vi "MNK_Dashboard_v2.vi"() -> ()   [LabVIEW 2013]
panel:
  out "magnet chart":dbl(graph)
  out "LN2 chart":dbl(graph)
  out "LHe chart":dbl(graph)
  out "temperature chart":dbl(graph)
  in  "Preferences Button":bool
  in  "OK":bool
  out "LN2 Level (mm)":dbl
  out "LHe Level (mm)":dbl
  out "Temperature (mK)":dbl format="%_3p"
  out "Magnetic Field (T)":dbl format="%.2f"
  # "magnetic field (T)"
  # "temperature (mK)"
  # "LHe level (mm)"
  # "LN2 level (mm)"
  # "hit \"enter\" to stop (on What Is)"
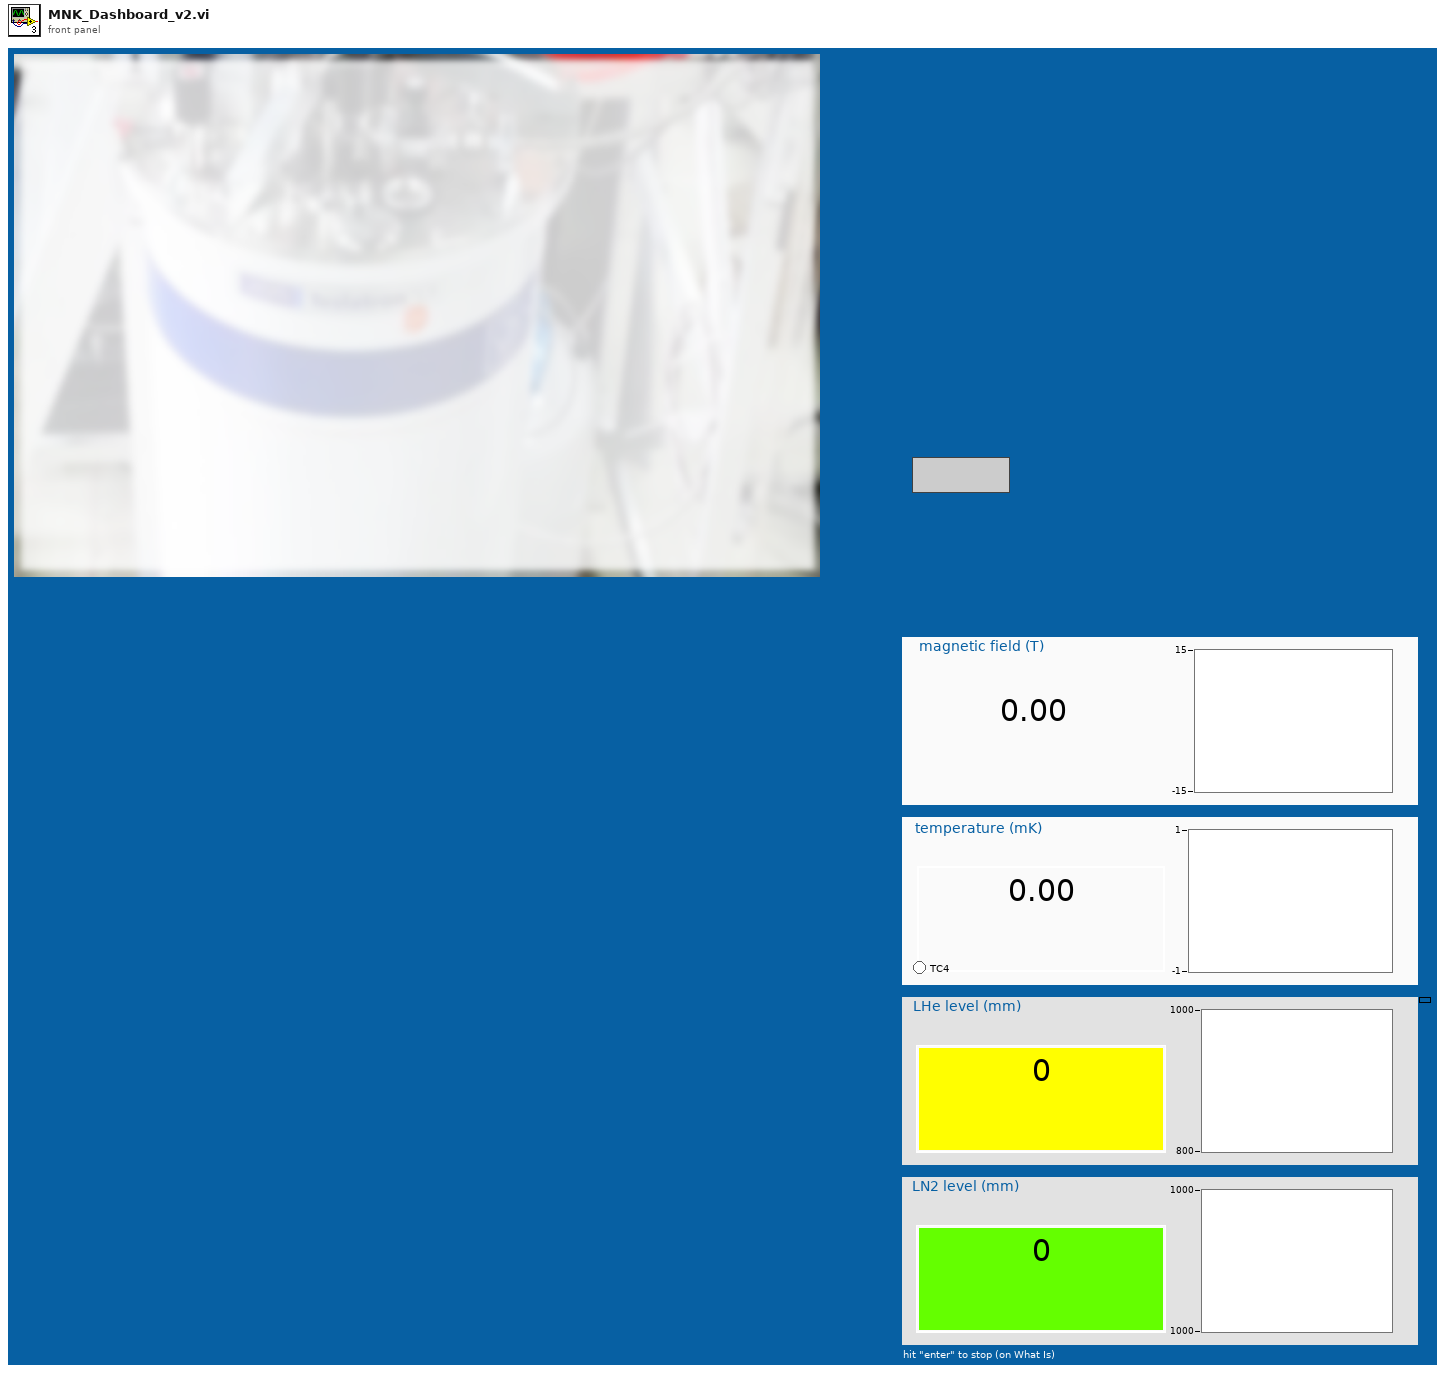
[diagram p1: front panel]
types:
  T1 = enum32{"invalid app kind", "Development System", "Run Time System", "Student Edition", "Embedded LabVIEW", "Evaluation", "Custom"}
  T2 = enum32{"Invalid", "Standard", "Closed", "Hidden", "Minimized", "Maximized"}
  T3 = cluster{"Core":cluster{"Current VI Reference":refnum<vi>, "Close Panel on Exit?":bool}, "Your Boolean data":bool, "Your string data":string}
  T4 = cluster{"Current VI Reference":refnum<vi>, "Close Panel on Exit?":bool}
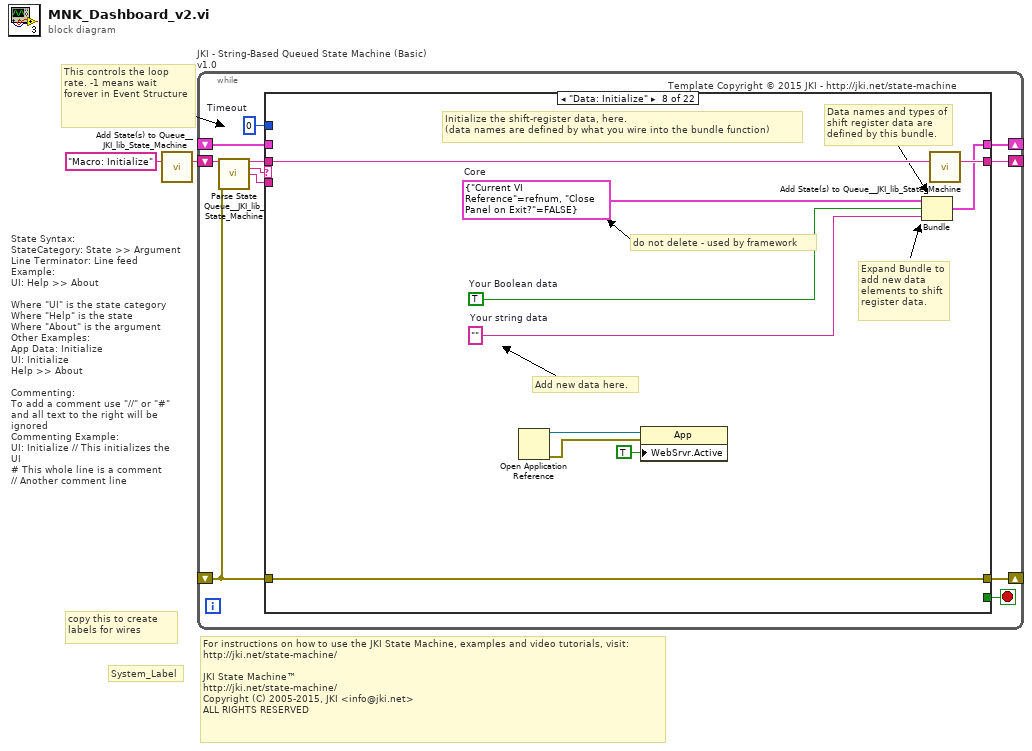
[diagram p0: block diagram]
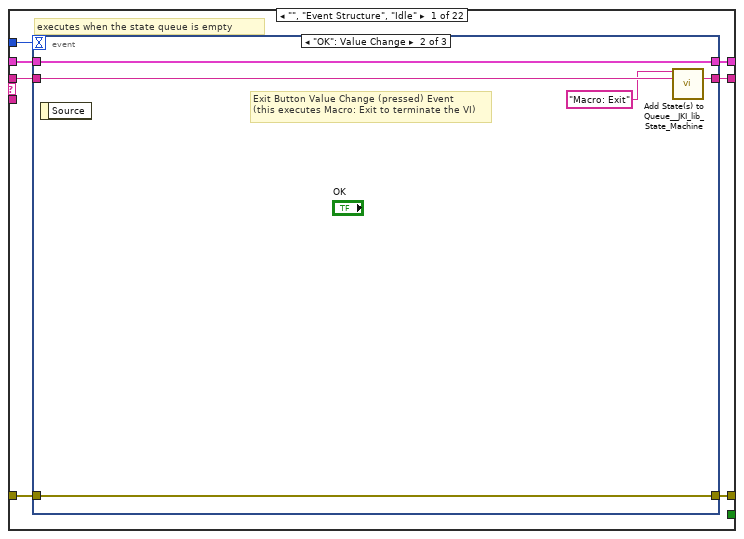
[diagram p2: hidden frame]
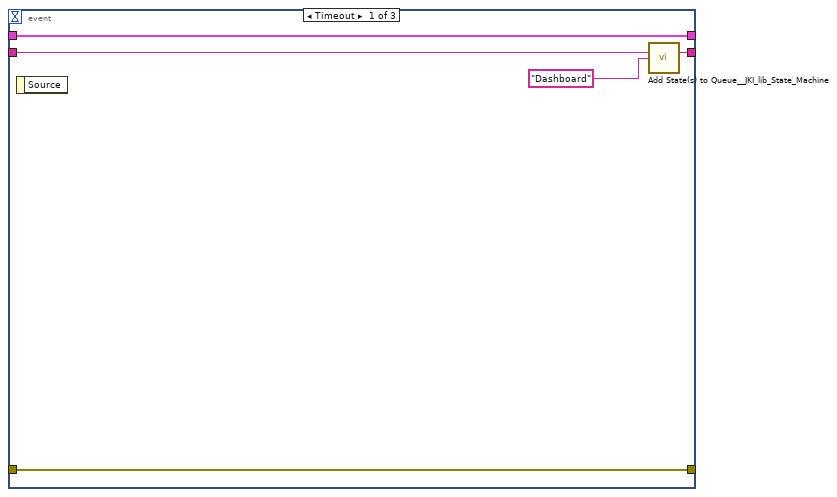
[diagram p3: hidden frame]
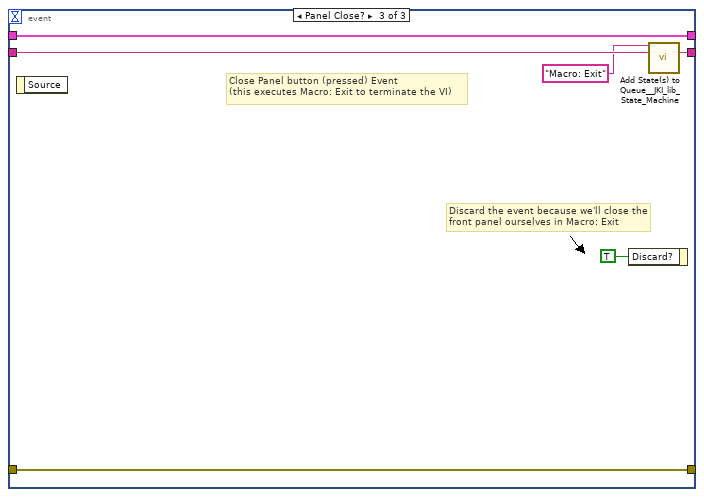
[diagram p4: hidden frame]
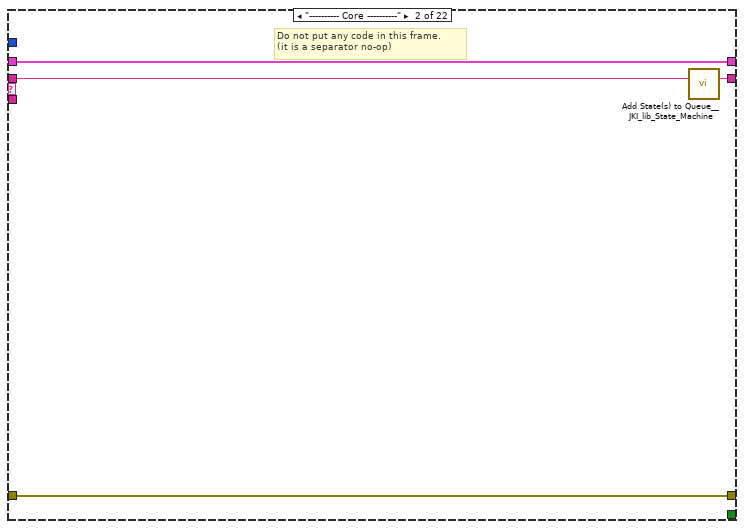
[diagram p5: hidden frame]
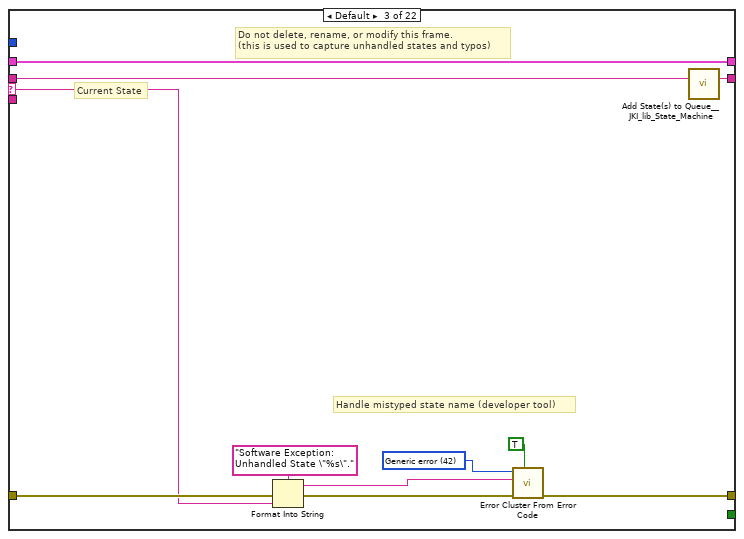
[diagram p6: hidden frame]
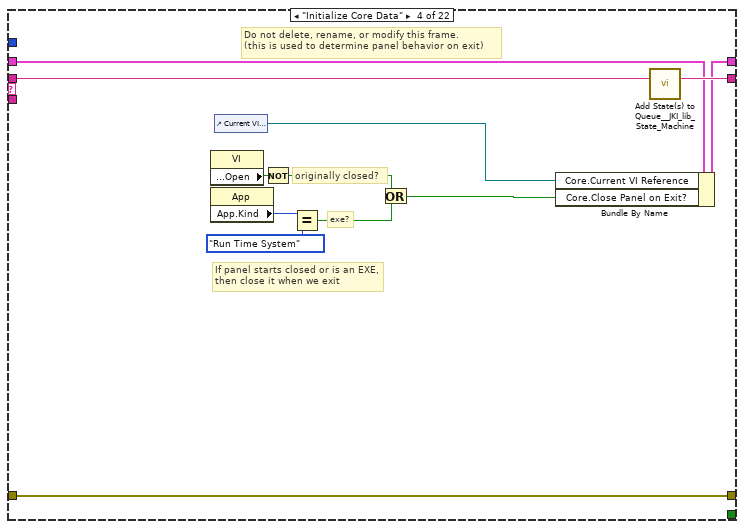
[diagram p7: hidden frame]
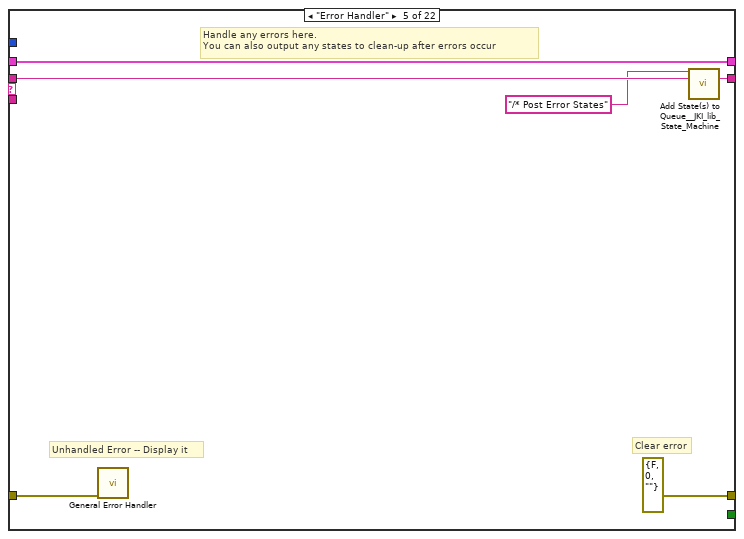
[diagram p8: hidden frame]
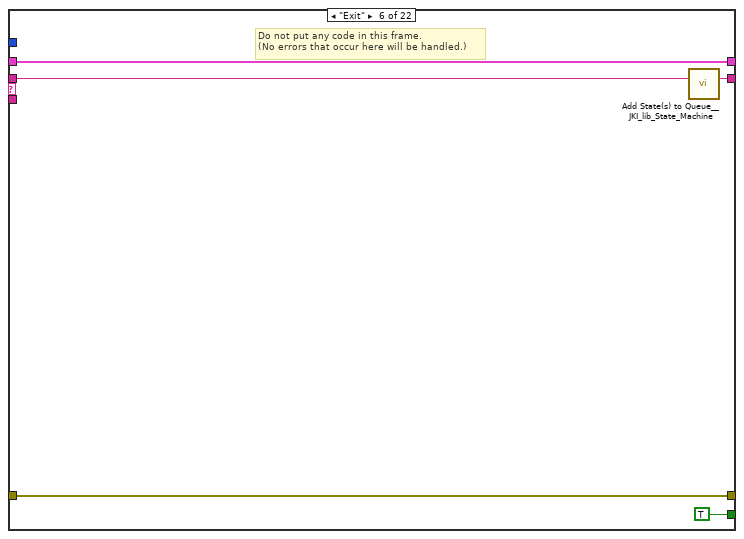
[diagram p9: hidden frame]
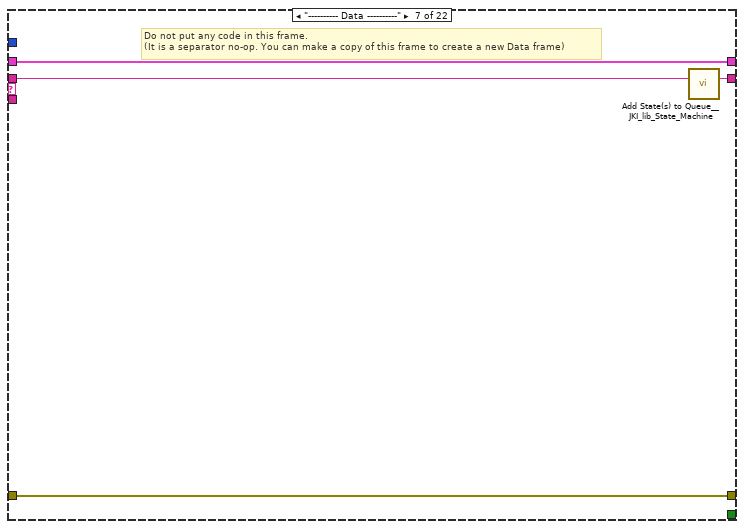
[diagram p10: hidden frame]
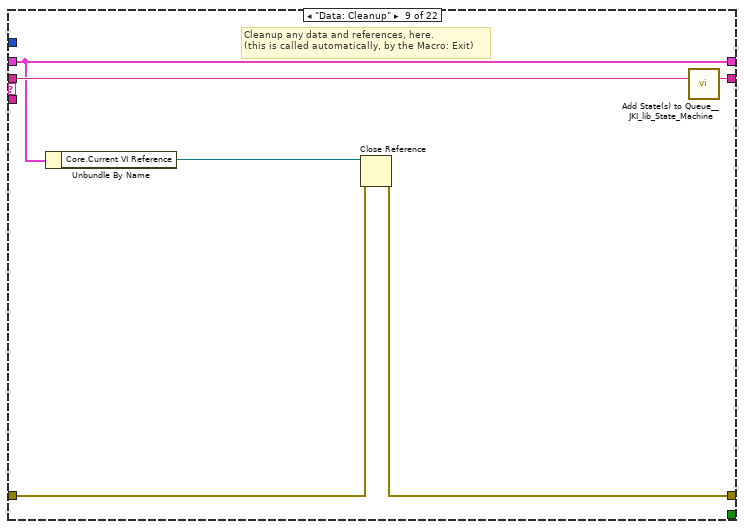
[diagram p11: hidden frame]
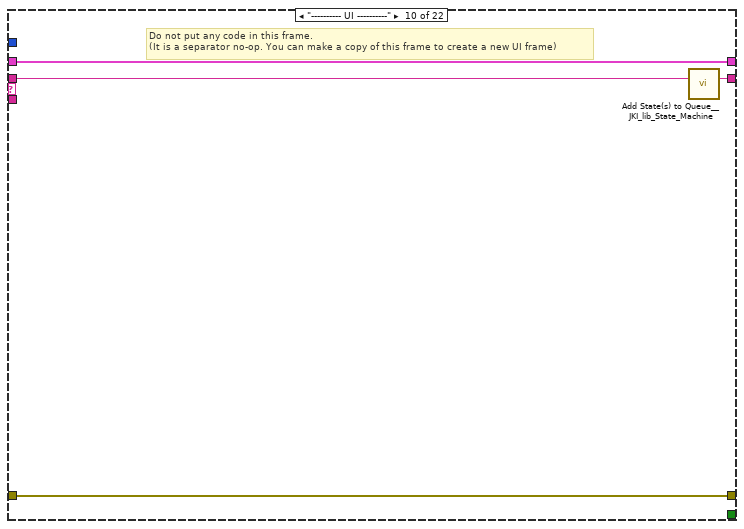
[diagram p12: hidden frame]
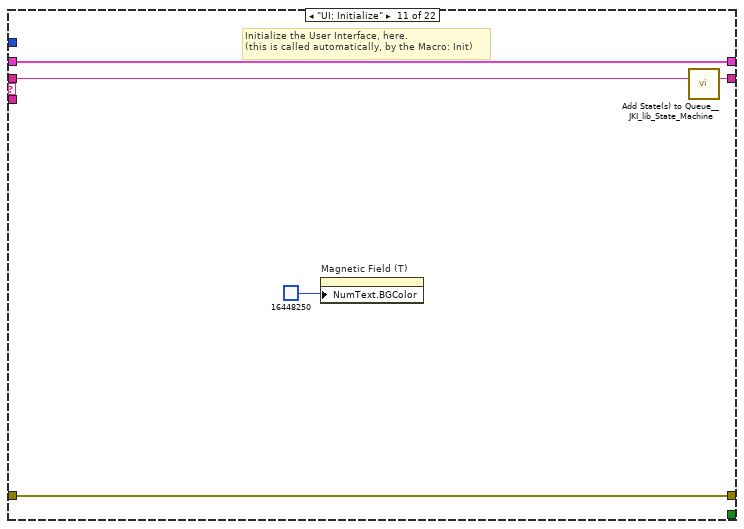
[diagram p13: hidden frame]
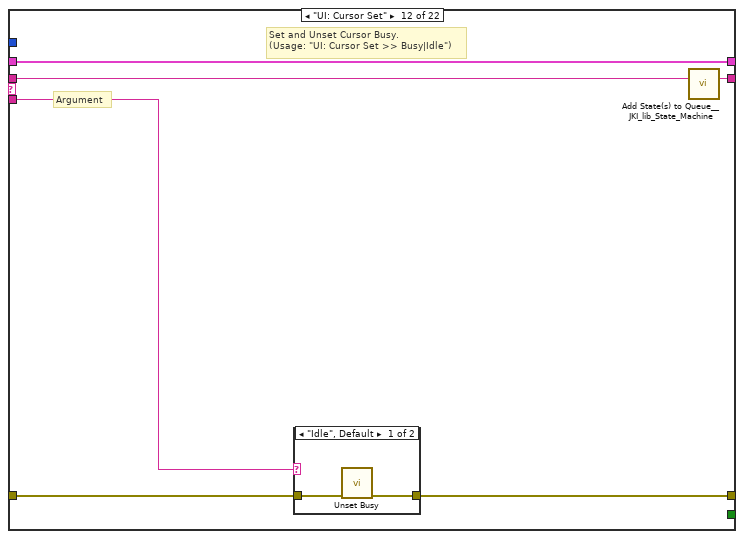
[diagram p14: hidden frame]
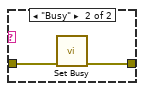
[diagram p15: hidden frame]
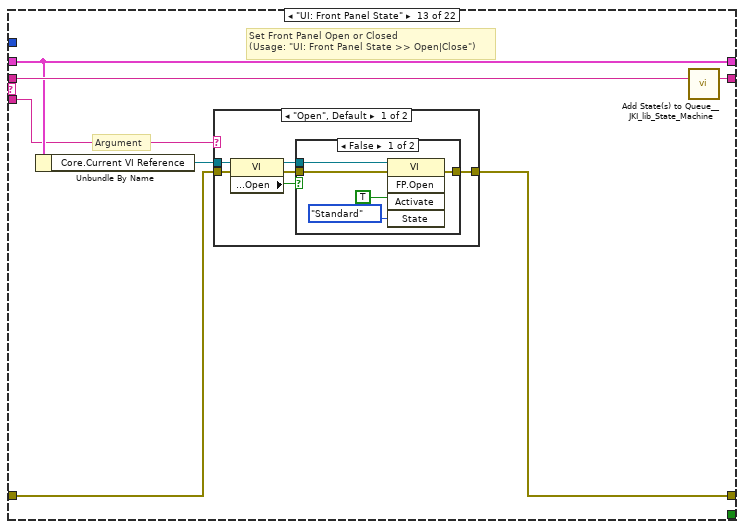
[diagram p16: hidden frame]
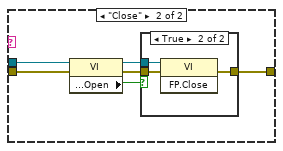
[diagram p18: hidden frame]
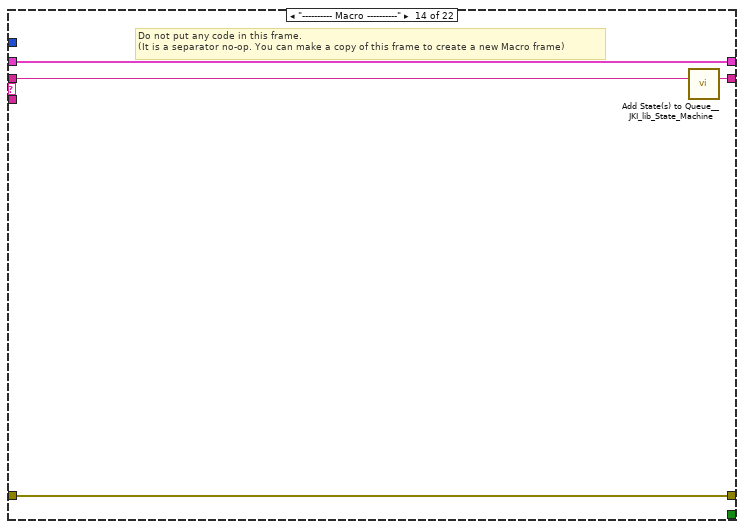
[diagram p20: hidden frame]
diagram:
  # "For instructions on how to use the JKI State Machine, examples and video tutorials, visit:\nhttp://jki.net/state-machine/\n\nJKI State Machine™\nhttp://jki.net/state-machine/\nCopyright (C) 2005-2015, JKI <info@jki.net>\nALL RIGHTS RESERVED"
  # "State Syntax:\nStateCategory: State >> Argument\nLine Terminator: Line feed\nExample:\nUI: Help >> About\n\nWhere \"UI\" is the state category\nWhere \"Help\" is the state\nWhere \"About\" is the argument\nOther Examples:\nApp Data: Initialize\nUI: Initialize\nHelp >> About\n\nCommenting:\nTo add a comment use \"//\" or \"#\" and all text to the right will be ignored\nCommenting Example:\nUI: Initialize // This initializes the UI\n# This whole line is a comment\n// Another comment line"
  # "copy this to create labels for wires"
  # "This controls the loop rate. -1 means wait forever in Event Structure"
  # "System_Label"
  n1 = call <vilib>:"Add State(s) to Queue__JKI_lib_State_Machine.vi"("State(s) in (\"\")"="Macro: Initialize") -> ("States Out"=w2:string)  [unwired: 14 in]
  n2 = while "JKI - String-Based Queued State Machine (Basic) v1.0" {
    shift-right: [w6] -> _
    shift-left: _ -> [w5]
    shift-right: [w9] -> _
    shift-left: _ -> [w3]
    shift-right: [w8] -> _
    shift-left: w2 -> [w10]
    stop <- w7 stop-if-true
    w4 = 0  # Timeout
    # "Template Copyright © 2015 JKI - http://jki.net/state-machine"
    n3 = call <vilib>:"Parse State Queue__JKI_lib_State_Machine.vi"("State Queue"=w10, "Error In (no error)"=w3) -> ("Remaining States"=w12:string, "Current State"=w13:string, "Arguments"=w11:string)  [unwired: 11 in]
    n4 = case shown="\"Data: Initialize\"" w13 {
      selector: w13 -> [_ _ w41 _ _ _ _ _ _ _ _ _ _ _ _ _ _ _ _ _ _ _]
      tunnel: w12 -> [w20 w40 w45 w63 w69 w74 w78 w88 w94 w98 w103 w109 w120 w146 w151 w161 w165 w170 w186 w199 w225 w241]
      tunnel: w11 -> [_ _ _ _ _ _ _ _ _ _ _ w104 w114 _ _ _ _ _ _ _ _ _]
      tunnel: w5 -> [w18 w37 w43 w54 w66 w72 w75 _ w89 w95 w101 w107 w116 w143 w148 w158 w162 w168 w184 w197 w223 w239]
      tunnel: [w17 w38 w47 w60 errorcluster {"status"=FALSE, "code"=0, "source"=""} ("error out") w71 w76 w85 w90 w96 w100 w105 w117 w144 w149 w159 w163 w167 w175 w188 w213 w228] -> w9
      tunnel: w3 -> [w16 w38 w46 w60 w65 w71 w76 w85 w91 w96 w100 w106 w118 w144 w149 w159 w163 w167 w174 w189 w212 w227]
      tunnel: [w19 w39 w44 w62 w68 w73 w77 w87 w93 w97 w102 w108 w119 w145 w150 w160 w164 w169 w185 w198 w224 w240] -> w8
      tunnel: [_ _ _ _ _ TRUE _ _ _ _ _ _ _ _ _ _ _ _ _ _ _ _] -> w7
      tunnel: [w15 w37 w43 w61 w66 w72 w75 w86 w89 w95 w101 w107 w116 w143 w148 w158 w162 w168 w184 w197 w223 w239] -> w6
      tunnel: w4 -> [w14 _ _ _ _ _ _ _ _ _ _ _ _ _ _ _ _ _ _ _ _ _]
      frame "", "Event Structure", "Idle" {
        # "executes when the state queue is empty"
        n5 = event shown="[1] \"OK\": Value Change" {
          selector: _ -> [_ _ _]
          dyn-events: _ -> [_ _ _]
          timeout: w14 -> [_ _ _]
          tunnel: w20 -> [w25 w30 w36]
          tunnel: [w24 w29 w35] -> w19
          tunnel: w18 -> [w23 w27 w33]
          tunnel: [w22 w28 w34] -> w17
          tunnel: w16 -> [w22 w28 w34]
          tunnel: [w23 w27 w33] -> w15
          event Timeout {
            n6 = event-data() -> ()  [unwired: 1 in, 1 out]
            n7 = call <vilib>:"Add State(s) to Queue__JKI_lib_State_Machine.vi"("State(s) in (\"\")"=w25, "State(s) at Back (\"\")"="Dashboard") -> ("States Out"=w24:string)  [unwired: 13 in]
          }
          event "OK": Value Change {
            # "Exit Button Value Change (pressed) Event\n(this executes Macro: Exit to terminate the VI)"
            n8 = event-data() -> ()  [unwired: 1 in, 1 out]
            n9 = call <vilib>:"Add State(s) to Queue__JKI_lib_State_Machine.vi"("State(s) in Front (\"\")"="Macro: Exit", "State(s) in (\"\")"=w30) -> ("States Out"=w29:string)  [unwired: 13 in]
          }
          event Panel Close? {
            # "Discard the event because we'll close the front panel ourselves in Macro: Exit"
            # "Close Panel button (pressed) Event\n(this executes Macro: Exit to terminate the VI)"
            n10 = event-data() -> ()  [unwired: 1 in, 1 out]
            n11 = event-data("Discard?"=TRUE) -> ()  [unwired: 1 in, 1 out]
            n12 = call <vilib>:"Add State(s) to Queue__JKI_lib_State_Machine.vi"("State(s) in Front (\"\")"="Macro: Exit", "State(s) in (\"\")"=w36) -> ("States Out"=w35:string)  [unwired: 13 in]
          }
        }
      }
      frame "---------- Core ----------" {
        # "Do not put any code in this frame.\n(it is a separator no-op)"
        n13 = call <vilib>:"Add State(s) to Queue__JKI_lib_State_Machine.vi"("State(s) in (\"\")"=w40) -> ("States Out"=w39:string)  [unwired: 14 in]
      }
      frame Default {
        w50 = 42 items=["No error", "Argument error", "Memory is full", "Out of zone", "End of file", "File already open", "Generic file I/O error", "File not found", "File permission error", "Disk is full", "Duplicate path", "Too many files open", "System feature not enabled", "Resource file not found", "Cannot add resource", "Resource not found", "Image not found", "Image memory error", "Pen does not exist", "Config type invalid", "Config token not found", "Config parse error", "Config memory error", "Bad external code format", "Bad external code offset", "External code not present", "Null window", "Destroy window error", "Null menu", "Print aborted", "Bad print record", "Print driver error", "Windows error during printing", "Memory error during printing", "Print dialog error", "Generic print error", "Invalid device refnum", "Device not found", "Device parameter error", "Device unit error", "Cannot open device", "Device call aborted", "Generic error", "Cancelled by user", "Object ID too low", "Object ID too high", "Object not in heap", "Unknown heap", "Unknown object (invalid DefProc)", "Unknown object (DefProc not in table)", "Message out of range", "Invalid (null) method", "Unknown message", "Manager call not supported", "Bad address", "Network operation in progress", "Network operation timed out", "Connection is busy", "Network attribute not supported", "Network error", "Address in use", "System out of memory", "Connection aborted", "Connection refused", "Not connected", "Already connected", "Connection closed", "Initialization error (interapplication manager)", "Bad occurrence", "Wait on unbound occurrence handler", "Occurrence queue overflow", "Datalog type conflict", "Unused", "Unrecognized type (interapplication manager)", "Memory corrupt", "Failed to make temporary DLL", "Old CIN version", "Drag socket not found", "Failed to load drop-object", "Failed to register OLE object", "Failed to release OLE object", "Format specifier type mismatch", "Unknown format specifier", "Too few format specifiers", "Too many format specifiers", "Scan failed", "Newer CIN version", "Error converting to variant", "Runtime menu error", "Password tampered", "Variant attribute not found", "Incompatible variant data type", "Event data is not available", "Event Store is not present", "Occurrence is not found", "Event Queue is not created", "Event info is not available", "Refnum passed is NULL", "Error retrieving Class GUID", "Error retrieving CoClass GUID", "Error retrieving TypeLib GUID.", "Bad built application magic bytes.", "Specific driver is different from the specific driver associated with the Logical Name.", "There is no session opened to the class driver.", "Max Error", "MAX - Error with config objects", "MAX - Error loading configuration", "MAX - Group not supported"]
        # "Current State"
        # "Do not delete, rename, or modify this frame.\n(this is used to capture unhandled states and typos)"
        # "Handle mistyped state name (developer tool)"
        n14 = Format Into String(format string="Software Exception: Unhandled State \"%s\"." ("message"), error in=w46, w41) -> (resulting string=w49:string, error out=w48:errorcluster)  [unwired: 1 in]
        n15 = call <vilib>:"Error Cluster From Error Code.vi"("show call chain? (False)"=TRUE, "error in (no error)"=w48, "error message (\"\")"=w49, "error code (0)"=w50) -> ("error out"=w47:errorcluster)  [unwired: 5 in]
        n16 = call <vilib>:"Add State(s) to Queue__JKI_lib_State_Machine.vi"("State(s) in (\"\")"=w45) -> ("States Out"=w44:string)  [unwired: 14 in]
      }
      frame "Initialize Core Data" {
        # "Do not delete, rename, or modify this frame.\n(this is used to determine panel behavior on exit)"
        # "originally closed?"
        # "exe?"
        # "If panel starts closed or is an EXE, then close it when we exit"
        n17 = property class="VI"() -> ("Front Panel.Open"=w59:bool)  [unwired: 2 in, 2 out]
        n18 = property class="App"() -> ("App.Kind"=w58:T1)  [unwired: 2 in, 2 out]
        n19 = control-ref of="Current VI Reference"() -> (w52:refnum<vi>)
        n20 = Not(x=w59) -> (.not. x?=w56:bool)
        n21 = Equal?(x=w58, y=T1."Run Time System" ("Application:Kind")) -> (x = y?=w55:bool)
        n22 = Or(x=w56, y=w55) -> (x .or. y?=w53:bool)
        n23 = Bundle By Name(cluster=w54, "Core.Current VI Reference"=w52, "Core.Close Panel on Exit?"=w53) -> (w61:T3)
        n24 = call <vilib>:"Add State(s) to Queue__JKI_lib_State_Machine.vi"("State(s) in (\"\")"=w63) -> ("States Out"=w62:string)  [unwired: 14 in]
      }
      frame "Error Handler" {
        # "Unhandled Error -- Display it"
        # "Handle any errors here.\nYou can also output any states to clean-up after errors occur"
        # "Clear error"
        n25 = call <vilib>:"General Error Handler.vi"("error in (no error)"=w65) -> ()  [unwired: 10 in, 5 out]
        n26 = call <vilib>:"Add State(s) to Queue__JKI_lib_State_Machine.vi"("State(s) in Front (\"\")"="/* Post Error States", "State(s) in (\"\")"=w69) -> ("States Out"=w68:string)  [unwired: 13 in]
      }
      frame "Exit" {
        # "Do not put any code in this frame.\n(No errors that occur here will be handled.)"
        n27 = call <vilib>:"Add State(s) to Queue__JKI_lib_State_Machine.vi"("State(s) in (\"\")"=w74) -> ("States Out"=w73:string)  [unwired: 14 in]
      }
      frame "---------- Data ----------" {
        # "Do not put any code in this frame.\n(It is a separator no-op. You can make a copy of this frame to create a new Data frame)"
        n28 = call <vilib>:"Add State(s) to Queue__JKI_lib_State_Machine.vi"("State(s) in (\"\")"=w78) -> ("States Out"=w77:string)  [unwired: 14 in]
      }
      frame "Data: Initialize" {
        w82 = T4 {"Current VI Reference"=refnum, "Close Panel on Exit?"=FALSE}  # Core
        w84 = TRUE  # Your Boolean data
        w83 = ""  # Your string data
        # "do not delete - used by framework"
        # "Expand Bundle to add new data elements to shift register data."
        # "Add new data here."
        # "Data names and types of shift register data are defined by this bundle."
        # "Initialize the shift-register data, here.\n(data names are defined by what you wire into the bundle function)"
        n29 = Open Application Reference() -> (0:w80:errorcluster, 3:w81:refnum<vi>)  [unwired: 4 in]
        n30 = property class="App"(reference=w81, error in=w80, "WebSrvr.Active"=TRUE ("Web Server:Server Active")) -> ()  [unwired: 2 out]
        n31 = Bundle("Core"=w82, "Your Boolean data"=w84, "Your string data"=w83) -> (w86:T3)  [unwired: 1 in]
        n32 = call <vilib>:"Add State(s) to Queue__JKI_lib_State_Machine.vi"("State(s) in (\"\")"=w88) -> ("States Out"=w87:string)  [unwired: 14 in]
      }
      frame "Data: Cleanup" {
        # "Cleanup any data and references, here.\n(this is called automatically, by the Macro: Exit)"
        n33 = Unbundle By Name(w89) -> ("Core.Current VI Reference"=w92:refnum<vi>)
        n34 = Close Reference(reference=w92, error in (no error)=w91) -> (error out=w90:errorcluster)
        n35 = call <vilib>:"Add State(s) to Queue__JKI_lib_State_Machine.vi"("State(s) in (\"\")"=w94) -> ("States Out"=w93:string)  [unwired: 14 in]
      }
      frame "---------- UI ----------" {
        # "Do not put any code in this frame.\n(It is a separator no-op. You can make a copy of this frame to create a new UI frame)"
        n36 = call <vilib>:"Add State(s) to Queue__JKI_lib_State_Machine.vi"("State(s) in (\"\")"=w98) -> ("States Out"=w97:string)  [unwired: 14 in]
      }
      frame "UI: Initialize" {
        # "Initialize the User Interface, here.\n(this is called automatically, by the Macro: Init)"
        n37 = property on="Magnetic Field (T)" class="DigNum (strict)"("NumText.BGColor"=u32 16448250) -> ()  [unwired: 2 in, 2 out]
        n38 = call <vilib>:"Add State(s) to Queue__JKI_lib_State_Machine.vi"("State(s) in (\"\")"=w103) -> ("States Out"=w102:string)  [unwired: 14 in]
      }
      frame "UI: Cursor Set" {
        # "Argument"
        # "Set and Unset Cursor Busy.\n(Usage: \"UI: Cursor Set >> Busy|Idle\")"
        n39 = case shown="\"Idle\", Default" w104 {
          tunnel: w106 -> [w111 w113]
          tunnel: [w110 w112] -> w105
          frame "Idle", Default {
            n40 = call <vilib>:"Unset Busy.vi"("error in (no error)"=w111) -> ("error out"=w110:errorcluster)  [unwired: 10 in]
          }
          frame "Busy" {
            n41 = call <vilib>:"Set Busy.vi"("error in (no error)"=w113) -> ("error out"=w112:errorcluster)  [unwired: 9 in, 1 out]
          }
        }
        n42 = call <vilib>:"Add State(s) to Queue__JKI_lib_State_Machine.vi"("State(s) in (\"\")"=w109) -> ("States Out"=w108:string)  [unwired: 14 in]
      }
      frame "UI: Front Panel State" {
        # "Argument"
        # "Set Front Panel Open or Closed\n(Usage: \"UI: Front Panel State >> Open|Close\")"
        n43 = Unbundle By Name(w116) -> ("Core.Current VI Reference"=w115:refnum<vi>)
        n44 = case shown="\"Open\", Default" w114 {
          tunnel: w118 -> [w124 w137]
          tunnel: [w126 w138] -> w117
          tunnel: w115 -> [w125 w135]
          frame "Open", Default {
            n45 = property class="VI"(reference=w125, error in=w124) -> (reference out=w122:refnum<vi>, error out=w123:errorcluster, "Front Panel.Open"=w121:bool)
            n46 = case shown="False" w121 {
              tunnel: [w129 w132] -> w126
              tunnel: w123 -> [w128 w132]
              tunnel: w122 -> [w127 _]
              frame False {
                n47 = invoke class="VI" method="FP.Open"(reference=w127, error in=w128, "Activate"=TRUE, "State"=T2."Standard") -> (error out=w129:errorcluster)  [unwired: 1 in, 4 out]
              }
              frame True {
              }
            }
          }
          frame "Close" {
            n48 = property class="VI"(reference=w135, error in=w137) -> (reference out=w134:refnum<vi>, error out=w136:errorcluster, "Front Panel.Open"=w133:bool)
            n49 = case shown="True" w133 {
              tunnel: [w139 w142] -> w138
              tunnel: w136 -> [w139 w141]
              tunnel: w134 -> [_ w140]
              frame False {
              }
              frame True {
                n50 = invoke class="VI" method="FP.Close"(reference=w140, error in=w141) -> (error out=w142:errorcluster)  [unwired: 1 in, 2 out]
              }
            }
          }
        }
        n51 = call <vilib>:"Add State(s) to Queue__JKI_lib_State_Machine.vi"("State(s) in (\"\")"=w120) -> ("States Out"=w119:string)  [unwired: 14 in]
      }
      frame "---------- Macro ----------" {
        # "Do not put any code in this frame.\n(It is a separator no-op. You can make a copy of this frame to create a new Macro frame)"
        n52 = call <vilib>:"Add State(s) to Queue__JKI_lib_State_Machine.vi"("State(s) in (\"\")"=w146) -> ("States Out"=w145:string)  [unwired: 14 in]
      }
      frame "Macro: Initialize" {
        w147 = "Data: Initialize\nInitialize Core Data\nUI: Initialize\nUI: Front Panel State >> Open\nDashboard"  # Data: Initialize Initialize Core Data UI: Initialize UI: Front Panel State >> Open Dashboard
        # "Initialization Macro\n(This is called once, when the VI starts)"
        n53 = call <vilib>:"Add State(s) to Queue__JKI_lib_State_Machine.vi"("State(s) in Front (\"\")"=w147, "State(s) in (\"\")"=w151) -> ("States Out"=w150:string)  [unwired: 13 in]
      }
      frame "Macro: Exit" {
        # "Exit Macro\n(This is called once, when the VI exits)"
        n54 = Unbundle By Name(w158) -> ("Core.Close Panel on Exit?"=w157:bool)
        n55 = Select(t="UI: Front Panel State >> Close", s=w157, f="") -> (s? t:f=w154:string)
        n56 = call <vilib>:"Add State(s) to Queue__JKI_lib_State_Machine.vi"("State(s) in (\"\")"=w154, "State(s) at Back (\"\")"="Data: Cleanup\nExit") -> ("States Out"=w152:string)  [unwired: 13 in]
        n57 = call <vilib>:"Add State(s) to Queue__JKI_lib_State_Machine.vi"("State(s) in Front (\"\")"=w152, "State(s) in (\"\")"=w161) -> ("States Out"=w160:string)  [unwired: 13 in]
      }
      frame "---------- Dashboard ----------" {
        # "Template Separator\n(You can make a copy of, or modify, this frame)"
        n58 = call <vilib>:"Add State(s) to Queue__JKI_lib_State_Machine.vi"("State(s) in (\"\")"=w165) -> ("States Out"=w164:string)  [unwired: 14 in]
      }
      frame "Dashboard" {
        n59 = call <vilib>:"Add State(s) to Queue__JKI_lib_State_Machine.vi"("State(s) in (\"\")"=w170, "State(s) at Back (\"\")"="Dashboard: temperature\nDashboard: magnet\nDashboard: LHe\nDashboard: LN2" ("State(s) at Back (\"\")")) -> ("States Out"=w169:string)  [unwired: 13 in]
      }
      frame "Dashboard: temperature" {
        n60 = Wait (ms)(milliseconds to wait=u32 100) -> ()  [unwired: 1 out]
        n61 = Select(t=refnum<k21> "ni.var.psp://housesoftheholy/MNK_18T/MNK_TC_T4" ("shared variable refnum in"), s="Preferences Button", f=refnum<k21> "ni.var.psp://housesoftheholy/MNK_18T/MNK_TC_T3" ("shared variable refnum in")) -> (s? t:f=w176:refnum<k21>)
        n62 = shared-variable-open(w176, w174, 0.0) -> (w182:refnum<k21>, w181:errorcluster)  [unwired: 1 in]
        n63 = shared-variable-read(w182, w181) -> (w179:refnum<k21>, w180:errorcluster, →"Temperature (mK)" →"temperature chart":dbl)  [unwired: 1 out]
        n64 = Close Variable Connection(8:w180, 11:w179) -> (0:w175:errorcluster)
        n65 = call <vilib>:"Add State(s) to Queue__JKI_lib_State_Machine.vi"("State(s) in (\"\")"=w186) -> ("States Out"=w185:string)  [unwired: 14 in]
      }
      frame "Dashboard: magnet" {
        n66 = shared-variable-open(refnum<k21> "ni.var.psp://housesoftheholy/MNK_18T/18T_Field" ("shared variable refnum in"), w189, 0.0) -> (w192:refnum<k21>, w193:errorcluster)  [unwired: 1 in]
        n67 = Wait (ms)(milliseconds to wait=u32 100) -> ()  [unwired: 1 out]
        n68 = shared-variable-read(w192, w193) -> (w195:refnum<k21>, w194:errorcluster, w187:dbl)  [unwired: 1 out]
        "Magnetic Field (T)" <- w187
        "magnet chart" <- w187
        n69 = Close Variable Connection(8:w194, 11:w195) -> (0:w188:errorcluster)
        n70 = disable-structure shown="Disabled" {
          frame Disabled {
            # "this code will make\nbg blink"
            n71 = property on="Magnetic Field (T)" class="DigNum (strict)"() -> ("NumText.BGColor"=w208:u32)  [unwired: 2 in, 2 out]
            n72 = Equal?(x=w208, y=u32 16448250) -> (x = y?=w207:bool)
            n73 = Select(t=u32 16719872, s=w207, f=u32 16448250) -> ()  [unwired: 1 out]
          }
          frame Enabled {
          }
        }
        n74 = disable-structure shown="Disabled" {
          disable-tunnel: w187 -> [w200 _]
          frame Disabled {
            n75 = Not Equal To 0?(x=w200) -> (x != 0?=w202:bool)
            n76 = Select(t=u32 16719872, s=w202, f=u32 16448250) -> (s? t:f=w204:u32)
            n77 = property on="Magnetic Field (T)" class="DigNum (strict)"("NumText.BGColor"=w204) -> ()  [unwired: 2 in, 2 out]
          }
          frame Enabled {
          }
        }
        n78 = call <vilib>:"Add State(s) to Queue__JKI_lib_State_Machine.vi"("State(s) in (\"\")"=w199) -> ("States Out"=w198:string)  [unwired: 14 in]
      }
      frame "Dashboard: LHe" {
        n79 = shared-variable-open(refnum<k21> "ni.var.psp://housesoftheholy/MNK_18T/18T_HeLevel" ("shared variable refnum in"), w212, 0.0) -> (w216:refnum<k21>, w217:errorcluster)  [unwired: 1 in]
        n80 = Wait (ms)(milliseconds to wait=u32 100) -> ()  [unwired: 1 out]
        n81 = shared-variable-read(w216, w217) -> (w219:refnum<k21>, w218:errorcluster, w210:dbl)  [unwired: 1 out]
        "LHe chart" <- w210
        n82 = Close Variable Connection(8:w218, 11:w219) -> (0:w213:errorcluster)
        n83 = control-ref of="LHe Level (mm)"() -> (w211:refnum<vi>)
        n84 = call "ColorIndicators_2Colors.vi"("Numeric"=w210, "alarm 1"=1100.0 ("y"), "alarm 2"=900.0 ("y"), "Digital in"=w211) -> ()  [unwired: 8 in]
        n85 = call <vilib>:"Add State(s) to Queue__JKI_lib_State_Machine.vi"("State(s) in (\"\")"=w225) -> ("States Out"=w224:string)  [unwired: 14 in]
      }
      frame "Dashboard: LN2" {
        w226 = 1200.0 ("Numeric")
        n86 = shared-variable-open(refnum<k21> "ni.var.psp://housesoftheholy/MNK_18T/18T_HeLevel" ("shared variable refnum in"), w227, 0.0) -> (w233:refnum<k21>, w232:errorcluster)  [unwired: 1 in]
        n87 = Wait (ms)(milliseconds to wait=u32 100) -> ()  [unwired: 1 out]
        n88 = shared-variable-read(w233, w232) -> (w230:refnum<k21>, w231:errorcluster)  [unwired: 2 out]
        n89 = Close Variable Connection(8:w231, 11:w230) -> (0:w228:errorcluster)
        n90 = control-ref of="LN2 Level (mm)"() -> (w229:refnum<vi>)
        n91 = call "ColorIndicators_2Colors.vi"("Numeric"=w226, "alarm 1"=1100.0 ("y"), "alarm 2"=900.0 ("y"), "Digital in"=w229) -> ()  [unwired: 8 in]
        n92 = call <vilib>:"Add State(s) to Queue__JKI_lib_State_Machine.vi"("State(s) in (\"\")"=w241) -> ("States Out"=w240:string)  [unwired: 14 in]
        "LN2 Level (mm)" <- w226
        "LN2 chart" <- w226
      }
    }
  }
